vi "Format String To Time Info.vi"(11 "Format String":string) -> (3 "Time Info":T1)   [LabVIEW 2018, in "Numeric Data Type.lvclass"]
uses:
  Numeric Data Type.lvclass
  Time Info.ctl
  Time Format.ctl
  Numeric Format Enum.ctl
  Clock Type.ctl
  Date Order.ctl
  Date Format.ctl
  Year Format.ctl
panel:
  # "(10 = Absolute)"
  # "0 = Local (No DST String)\n1 = UTC (No DST String)\n2 = Local (With DST String)\n3 = UTC (With DST String)"
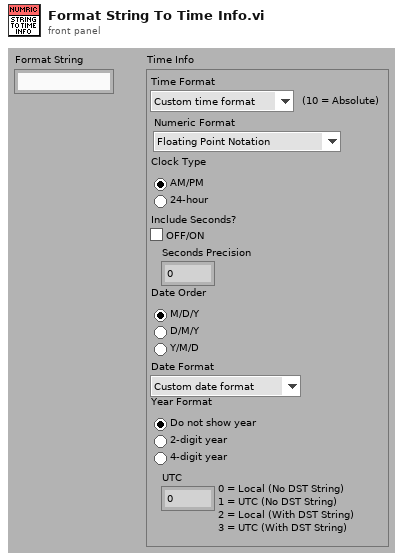
[diagram p1: front panel]
types:
  T1 = typedef "Numeric Data Type.lvclass/Time Info.ctl" = cluster{"Time Format":T2, "Numeric Format":T3, "Clock Type":T4, "Include Seconds?":bool, "Seconds Precision":i16, "Date Order":T5, "Date Format":T6, "Year Format":T7, "UTC":i16}
  T2 = typedef "Numeric Data Type.lvclass/Time Format.ctl" = enum16{"Custom time format", "System time format", "Time unused"}
  T3 = typedef "Numeric Data Type.lvclass/Numeric Format Enum.ctl" = enum16{"Floating Point Notation", "Scientific Notation", "Engineering Notation", "SI Notation", "<not used>", "Decimal", "Hexadecimal", "Octal", "Binary", "<not used 2>", "Absolute Time", "Relative Time"}
  T4 = typedef "Numeric Data Type.lvclass/Clock Type.ctl" = enum32{"12-Hour (AM/PM)", "24-Hour"}
  T5 = typedef "Numeric Data Type.lvclass/Date Order.ctl" = enum32{"M/D/Y", "D/M/Y", "Y/M/D"}
  T6 = typedef "Numeric Data Type.lvclass/Date Format.ctl" = enum16{"Custom date format", "System date format", "Date unused"}
  T7 = typedef "Numeric Data Type.lvclass/Year Format.ctl" = enum32{"No Year", "2-digit Year", "4-digit Year"}
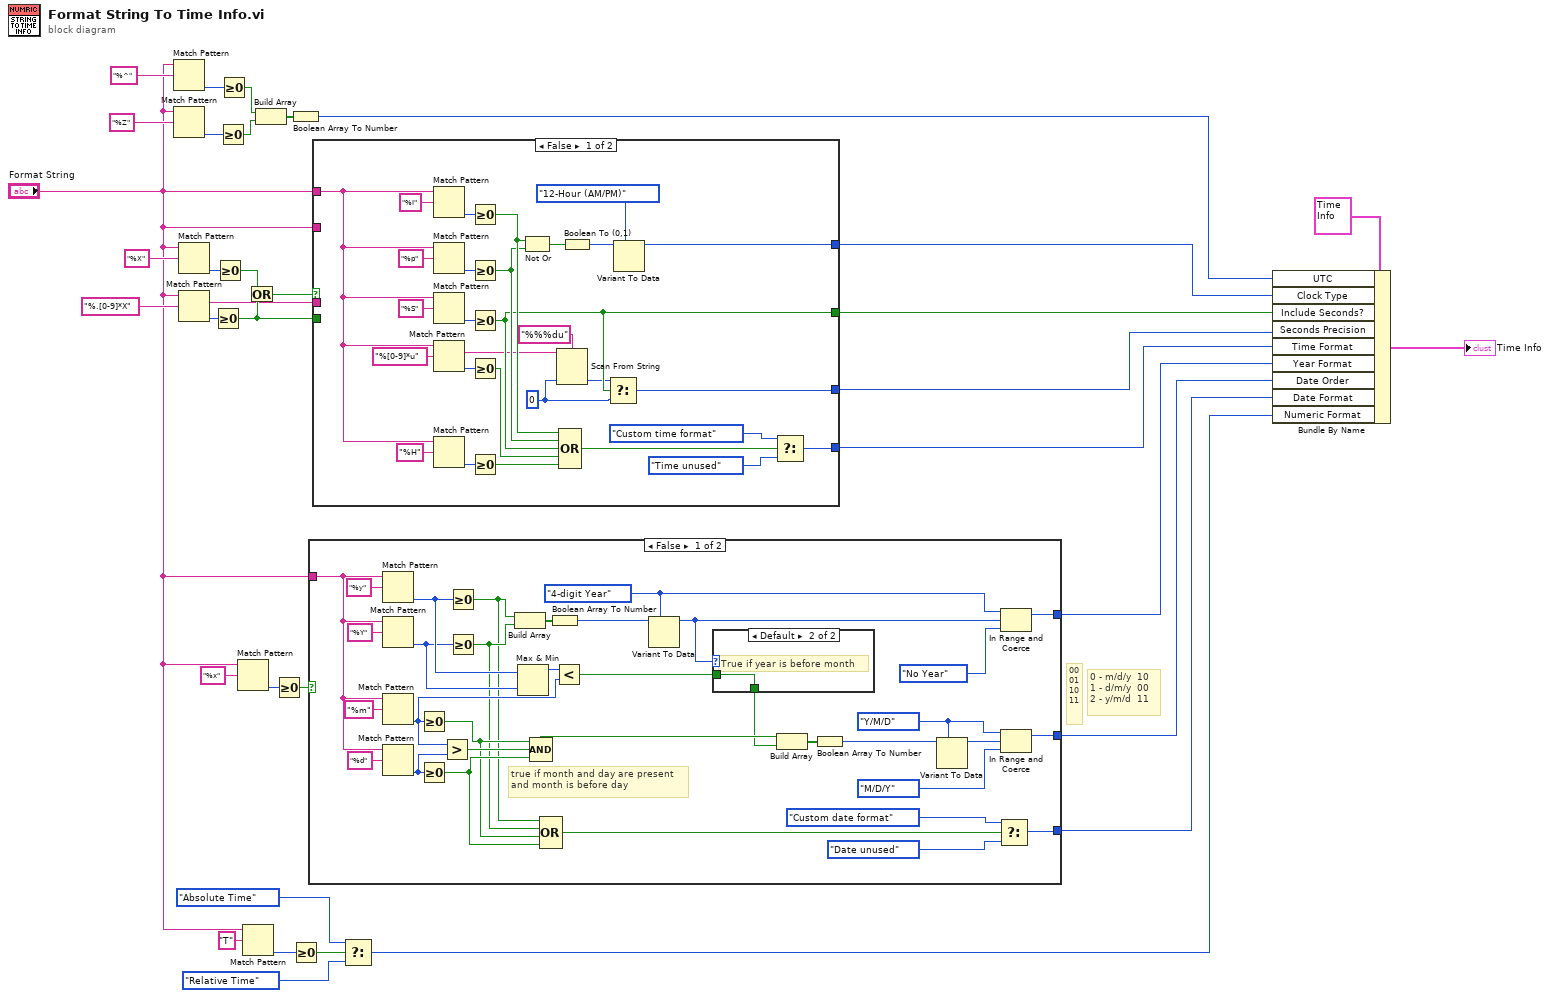
[diagram p0: block diagram]
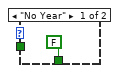
[diagram p2: hidden frame]
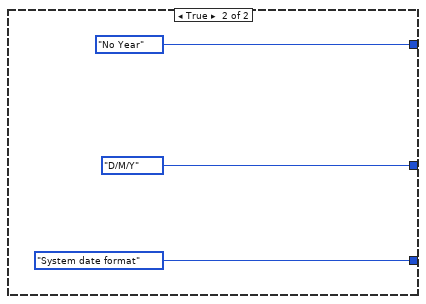
[diagram p3: hidden frame]
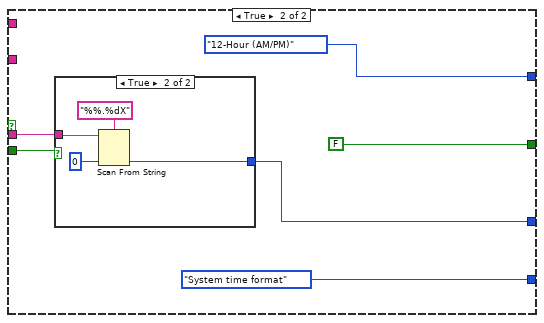
[diagram p4: hidden frame]
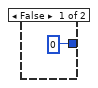
[diagram p5: hidden frame]
diagram:
  # "0 - m/d/y  10\n1 - d/m/y  00\n2 - y/m/d  11"
  # "00\n01\n10\n11"
  n1 = Match Pattern(string="Format String", regular expression="%^") -> (offset past match=w23:i32)  [unwired: 1 in, 3 out]
  n2 = Match Pattern(string="Format String", regular expression="%Z") -> (offset past match=w21:i32)  [unwired: 1 in, 3 out]
  n3 = Match Pattern(string="Format String", regular expression="%X") -> (offset past match=w35:i32)  [unwired: 1 in, 3 out]
  n4 = Match Pattern(string="Format String", regular expression="%.[0-9]*X") -> (match substring=w25:string, offset past match=w29:i32)  [unwired: 1 in, 2 out]
  n5 = Greater Or Equal To 0?(x=w29) -> (x >= 0?=w26:bool)
  n6 = Greater Or Equal To 0?(x=w35) -> (x >= 0?=w28:bool)
  n7 = Greater Or Equal To 0?(x=w21) -> (x >= 0?=w18:bool)
  n8 = Greater Or Equal To 0?(x=w23) -> (x >= 0?=w19:bool)
  n9 = Match Pattern(string="Format String", regular expression="%x") -> (offset past match=w32:i32)  [unwired: 1 in, 3 out]
  n10 = Match Pattern(string="Format String", regular expression="T") -> (offset past match=w9:i32)  [unwired: 1 in, 3 out]
  n11 = Or(x=w28, y=w26) -> (x .or. y?=w27:bool)
  n12 = Build Array(w19, w18) -> (w20:bool[])
  n13 = Greater Or Equal To 0?(x=w32) -> (x >= 0?=w31:bool)
  n14 = Boolean Array To Number(Boolean array=w20) -> (number=w16:u32)
  n15 = Greater Or Equal To 0?(x=w9) -> (x >= 0?=w8:bool)
  n16 = case shown="False" w31 {
    tunnel: "Format String" -> [w64 _]
    tunnel: [w62 Year_Format."No Year" ("Year Format")] -> w14
    tunnel: [w54 Date_Order."D/M/Y" ("Date Order")] -> w13
    tunnel: [w48 Date_Format."System date format" ("Date Format")] -> w3
    frame False {
      w39 = Date_Order."Y/M/D" ("Date Order")
      w44 = Year_Format."4-digit Year" ("Year Format")
      # "true if month and day are present\nand month is before day"
      n17 = Match Pattern(string=w64, regular expression="%y") -> (offset past match=w60:i32)  [unwired: 1 in, 3 out]
      n18 = Match Pattern(string=w64, regular expression="%Y") -> (offset past match=w59:i32)  [unwired: 1 in, 3 out]
      n19 = Match Pattern(string=w64, regular expression="%m") -> (offset past match=w57:i32)  [unwired: 1 in, 3 out]
      n20 = Match Pattern(string=w64, regular expression="%d") -> (offset past match=w65:i32)  [unwired: 1 in, 3 out]
      n21 = Greater Or Equal To 0?(x=w57) -> (x >= 0?=w52:bool)
      n22 = Greater Or Equal To 0?(x=w65) -> (x >= 0?=w53:bool)
      n23 = Greater?(x=w57, y=w65) -> (0:w61:bool)
      n24 = Greater Or Equal To 0?(x=w60) -> (x >= 0?=w50:bool)
      n25 = Greater Or Equal To 0?(x=w59) -> (x >= 0?=w51:bool)
      n26 = Build Array(w50, w51) -> (w63:bool[])
      n27 = Max & Min(x=w60, y=w59) -> (max(x,y)=w58:i32)  [unwired: 1 out]
      n28 = Compound Arithmetic op=AND(w52, w61, w53) -> (w55:bool)
      n29 = Compound Arithmetic op=OR(w50, w51, w52, w53) -> (w49:bool)
      n30 = Boolean Array To Number(Boolean array=w63) -> (number=w43:u32)
      n31 = Less?(x=w58, y=w57) -> (x < y?=w46:bool)
      n32 = Variant To Data(type=w44, Variant=w43) -> (data=w42:T7)  [unwired: 1 in, 1 out]
      n33 = case shown="Default" w42 {
        tunnel: [FALSE w71] -> w47
        tunnel: w46 -> [_ w71]
        frame "No Year" {
        }
        frame Default {
          # "True if year is before month"
        }
      }
      n34 = Build Array(w55, w47) -> (w56:bool[])
      n35 = Boolean Array To Number(Boolean array=w56) -> (number=w41:u32)
      n36 = Variant To Data(type=w39, Variant=w41) -> (data=w40:T5)  [unwired: 1 in, 1 out]
      n37 = Select(t=Date_Format."Custom date format" ("Date Format"), s=w49, f=Date_Format."Date unused" ("Date Format")) -> (s? t:f=w48:T6)
      n38 = In Range and Coerce(upper limit=w44, x=w42, lower limit=Year_Format."No Year" ("Year Format")) -> (coerced(x)=w62:T7)  [unwired: 1 out]
      n39 = In Range and Coerce(upper limit=w39, x=w40, lower limit=Date_Order."M/D/Y" ("Date Order")) -> (coerced(x)=w54:T5)  [unwired: 1 out]
    }
    frame True {
    }
  }
  n40 = case shown="False" w27 {
    tunnel: "Format String" -> [w84 _]
    tunnel: [w91 Time_Format."System time format" ("Time Format")] -> w4
    tunnel: [w78 Clock_Type."12-Hour (AM/PM)" ("Clock Type")] -> w5
    tunnel: [w88 FALSE] -> w6
    tunnel: [w87 w107] -> w15
    tunnel: "Format String" -> [_ _]
    tunnel: w26 -> [_ w109]
    tunnel: w25 -> [_ w108]
    frame False {
      w82 = i16 0 ("f")
      n41 = Match Pattern(string=w84, regular expression="%I") -> (offset past match=w101:i32)  [unwired: 1 in, 3 out]
      n42 = Match Pattern(string=w84, regular expression="%p") -> (offset past match=w100:i32)  [unwired: 1 in, 3 out]
      n43 = Match Pattern(string=w84, regular expression="%S") -> (offset past match=w99:i32)  [unwired: 1 in, 3 out]
      n44 = Match Pattern(string=w84, regular expression="%[0-9]*u") -> (match substring=w79:string, offset past match=w96:i32)  [unwired: 1 in, 2 out]
      n45 = Match Pattern(string=w84, regular expression="%H") -> (offset past match=w86:i32)  [unwired: 1 in, 3 out]
      n46 = Greater Or Equal To 0?(x=w101) -> (x >= 0?=w95:bool)
      n47 = Greater Or Equal To 0?(x=w100) -> (x >= 0?=w94:bool)
      n48 = Greater Or Equal To 0?(x=w99) -> (x >= 0?=w88:bool)
      n49 = Greater Or Equal To 0?(x=w96) -> (x >= 0?=w93:bool)
      n50 = Greater Or Equal To 0?(x=w86) -> (x >= 0?=w83:bool)
      n51 = Not Or(1:w94, 2:w95) -> (0:w90:bool)
      n52 = Scan From String(format string="%%%du", input string=w79, default 1=w82) -> (output 1=w81:i16)  [unwired: 2 in, 3 out]
      n53 = Compound Arithmetic op=OR(w95, w94, w88, w93, w83) -> (w92:bool)
      n54 = Boolean To (0,1)(Boolean=w90) -> (0, 1=w89:i16)
      n55 = Select(t=w81, s=w88, f=w82) -> (s? t:f=w87:i16)
      n56 = Variant To Data(type=Clock_Type."12-Hour (AM/PM)" ("Clock Type"), Variant=w89) -> (data=w78:T4)  [unwired: 1 in, 1 out]
      n57 = Select(t=Time_Format."Custom time format" ("Time Format"), s=w92, f=Time_Format."Time unused" ("Time Format")) -> (s? t:f=w91:T2)
    }
    frame True {
      n58 = case shown="True" w109 {
        tunnel: w108 -> [_ w114]
        tunnel: [i16 0 w112] -> w107
        frame False {
        }
        frame True {
          n59 = Scan From String(format string="%%.%dX", input string=w114, default 1=i16 0 ("default value 1")) -> (output 1=w112:i16)  [unwired: 2 in, 3 out]
        }
      }
    }
  }
  n60 = Select(t=Numeric_Format_Enum."Absolute Time" ("Numeric Format (Time is 10 OR 11)"), s=w8, f=Numeric_Format_Enum."Relative Time" ("Numeric Format (Time is 10 OR 11)")) -> (s? t:f=w7:T3)
  n61 = Bundle By Name(cluster=T1 {"Time Format"=enum."Custom time format", "Numeric Format"=enum."Floating Point Notation", "Clock Type"=enum."12-Hour (AM/PM)", "Include Seconds?"=FALSE, "Seconds Precision"=0, "Date Order"=enum."M/D/Y", "Date Format"=enum."Custom date format", "Year Format"=enum."No Year", "UTC"=0} ("Time Format & Precision Info"), "UTC"=w16, "Clock Type"=w5, "Include Seconds?"=w6, "Seconds Precision"=w15, "Time Format"=w4, "Year Format"=w14, "Date Order"=w13, "Date Format"=w3, "Numeric Format"=w7) -> (→"Time Info":T1)
